vi "Buffer write test.vi"() -> ()   [LabVIEW 2015]
panel:
  out "Boolean":bool=TRUE
  out "Buffer out 3":dbl[](array[numeric])
  out "subarray":dbl[](array[numeric])
  out "x-y*floor(x/y)":i32
  out "Buffer out 2":dbl[](array[numeric])
  in  "Index":i32
  out "Buffer out":dbl[](array[numeric])
  in  "Data":dbl[](array[numeric])
  in  "Buffer in":dbl[](array[numeric])
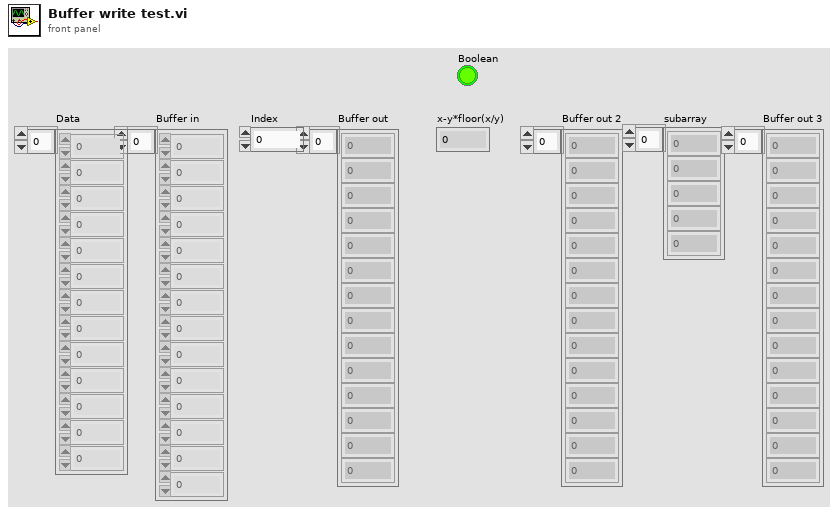
[diagram p1: front panel]
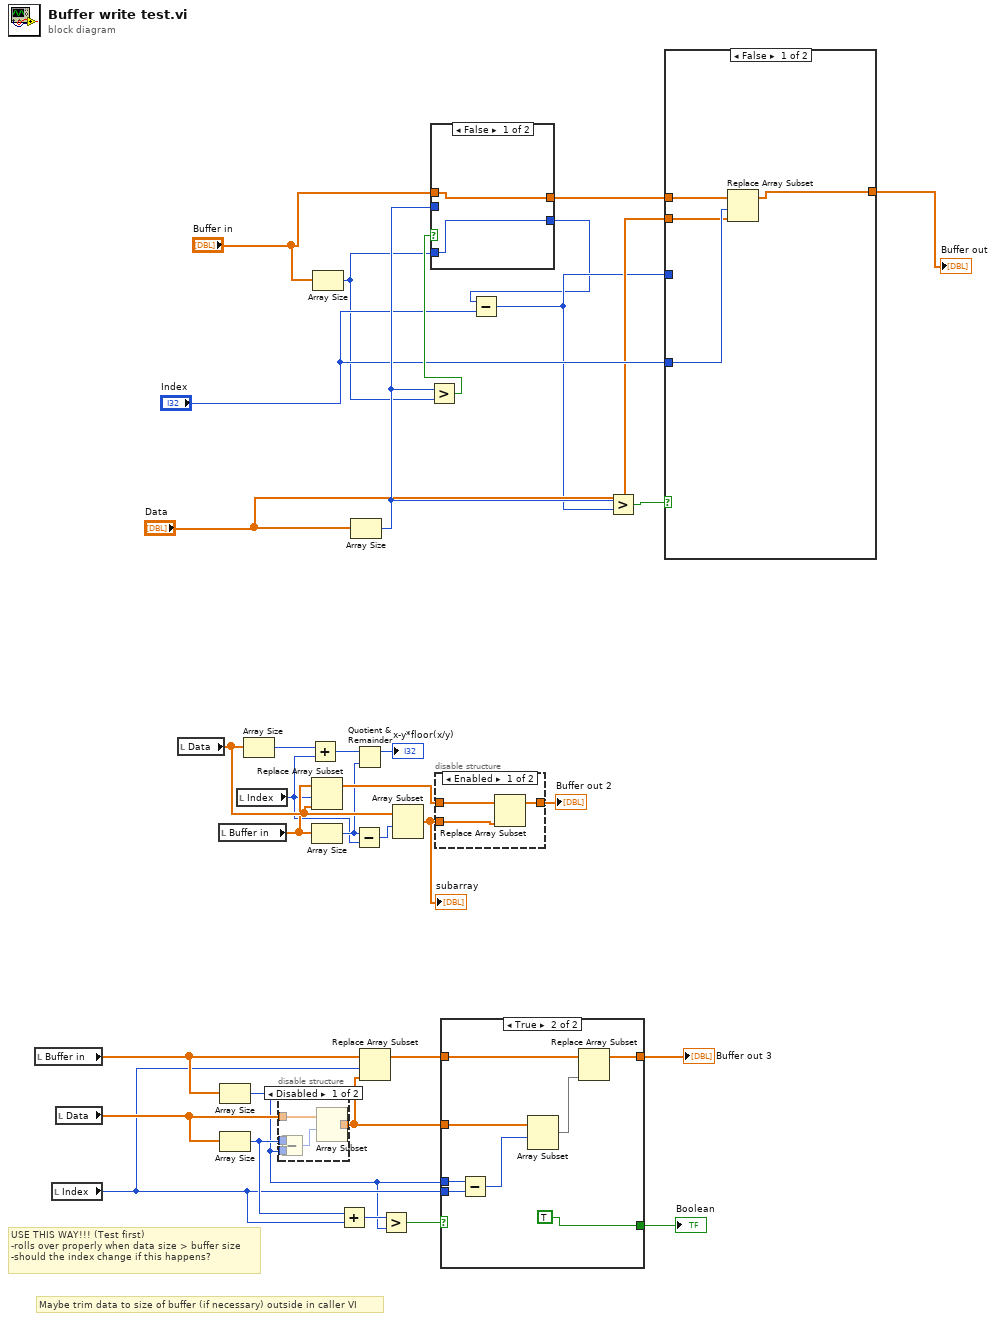
[diagram p0: block diagram]
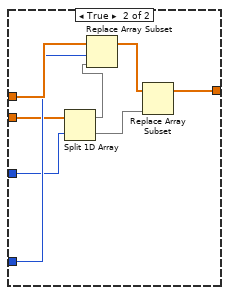
[diagram p5: hidden frame]
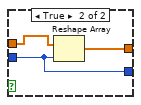
[diagram p6: hidden frame]
diagram:
  # "Maybe trim data to size of buffer (if necessary) outside in caller VI"
  # "USE THIS WAY!!! (Test first)\n-rolls over properly when data size > buffer size\n-should the index change if this happens?"
  n1 = local read "Buffer in"() -> (w10:dbl[])
  n2 = local read "Index"() -> (w5:i32)
  n3 = local read "Data"() -> (w8:dbl[])
  n4 = local read "Data"() -> (w21:dbl[])
  n5 = local read "Buffer in"() -> (w19:dbl[])
  n6 = Array Size(array=w10) -> (size(s)=w3:i32)
  n7 = Array Size(array=w8) -> (size(s)=w6:i32)
  n8 = local read "Index"() -> (w12:i32)
  n9 = Array Size(array=w21) -> (size(s)=w20:i32)
  n10 = disable-structure shown="Disabled" {
    disable-tunnel: w8 -> [w38 w39]
    disable-tunnel: w6 -> [w37 _]
    disable-tunnel: w3 -> [w36 _]
    disable-tunnel: [w34 w39] -> w7
    frame Disabled {
      n11 = Subtract(x=w37, y=w36) -> (x-y=w35:i32)
      n12 = Array Subset(array=w38, index=w35) -> (w34:dbl[])  [unwired: 1 in]
    }
    frame Enabled {
    }
  }
  n13 = Add(x=w20, y=w12) -> (x+y=w15:i32)
  n14 = Replace Array Subset(array=w19, new element=w21, index=w12) -> (w22:dbl[])
  n15 = Array Size(array=w19) -> (size(s)=w13:i32)
  n16 = Array Size(array="Buffer in") -> (size(s)=w24:i32)
  n17 = Add(x=w6, y=w5) -> (x+y=w4:i32)
  n18 = Array Size(array="Data") -> (size(s)=w31:i32)
  n19 = Subtract(x=w13, y=w12) -> (x-y=w14:i32)
  n20 = Quotient & Remainder(x=w15, y=w13) -> (x-y*floor(x/y)=→"x-y*floor(x/y)":i32)  [unwired: 1 out]
  n21 = Replace Array Subset(array=w10, new element=w7, index=w5) -> (w9:dbl[])
  n22 = Greater?(x=w4, y=w3) -> (0:w2:bool)
  n23 = Array Subset(array=w21, index=w14) -> (w18:dbl[])  [unwired: 1 in]
  "subarray" <- w18
  n24 = Greater?(x=w31, y=w24) -> (0:w33:bool)
  n25 = case shown="False" w33 {
    tunnel: "Buffer in" -> [w41 w44]
    tunnel: w31 -> [_ w42]
    tunnel: [w41 w43] -> w29
    tunnel: [w40 w42] -> w23
    tunnel: w24 -> [w40 _]
    frame False {
    }
    frame True {
      n26 = Reshape Array(w44, w42) -> (w43:dbl[])
    }
  }
  n27 = disable-structure shown="Enabled" {
    disable-tunnel: w22 -> [w47 w48]
    disable-tunnel: w18 -> [w46 _]
    disable-tunnel: [w45 w48] -> w17
    frame Enabled {
      n28 = Replace Array Subset(array=w47, new element=w46) -> (w45:dbl[])  [unwired: 1 in]
    }
    frame Disabled {
    }
  }
  "Buffer out 2" <- w17
  n29 = case shown="True" w2 {
    tunnel: w5 -> [_ w57]
    tunnel: [w49 w55] -> w11
    tunnel: w9 -> [w49 w53]
    tunnel: w3 -> [_ w52]
    tunnel: w7 -> [_ w51]
    tunnel: [_ TRUE] -> w1
    frame False {
    }
    frame True {
      n30 = Subtract(x=w52, y=w57) -> (x-y=w56:i32)
      n31 = Array Subset(array=w51, index=w56) -> (w54:dbl[])  [unwired: 1 in]
      n32 = Replace Array Subset(array=w53, new element=w54) -> (w55:dbl[])  [unwired: 1 in]
    }
  }
  "Buffer out 3" <- w11
  "Boolean" <- w1
  n33 = Subtract(x=w23, y="Index") -> (x-y=w26:i32)
  n34 = Greater?(x=w31, y=w26) -> (0:w30:bool)
  n35 = case shown="False" w30 {
    tunnel: w29 -> [w61 w69]
    tunnel: "Index" -> [w60 w68]
    tunnel: "Data" -> [w59 w66]
    tunnel: w26 -> [_ w65]
    tunnel: [w58 w62] -> w25
    frame False {
      n36 = Replace Array Subset(array=w61, new element=w59, index=w60) -> (w58:dbl[])
    }
    frame True {
      n37 = Split 1D Array(array=w66, index=w65) -> (first subarray=w64:dbl[], second subarray=w63:dbl[])
      n38 = Replace Array Subset(array=w69, new element=w64, index=w68) -> (w67:dbl[])
      n39 = Replace Array Subset(array=w67, new element=w63) -> (w62:dbl[])  [unwired: 1 in]
    }
  }
  "Buffer out" <- w25
